vi "Close.vi"(11 "Custom Device Utility in":refnum<class "Custom Device Utility.lvclass">) -> (0 "error out":errorcluster, 3 "Custom Device Utility out":refnum<class "Custom Device Utility.lvclass">)   [LabVIEW 2027, in "Custom Device Interfaces.lvlib" / "Custom Device Utility.lvclass"]
uses:
  Custom Device Utility.lvclass
  Custom Device Utility.lvclass/Custom Device Utility.ctl
  CustomDevice/Custom Device.lvclass
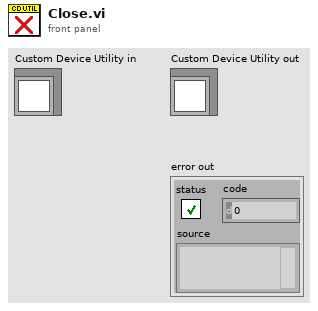
[diagram p1: front panel]
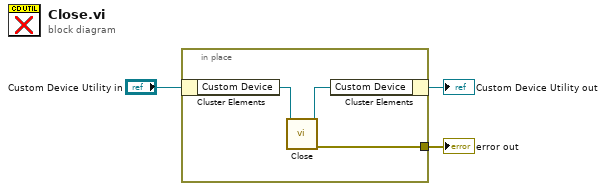
[diagram p0: block diagram]
diagram:
  n1 = in-place {
    in-place-border: [w6] -> w3
    n2 = in-place-cluster #1("Custom Device Utility in") -> ("Custom Device"=w5:refnum<class "Custom Device.lvclass">)
    n3 = call-dynamic "Close.vi"("Custom Device in"=w5) -> ("error out"=w6:errorcluster, "Custom Device out"=w4:refnum<class "Custom Device.lvclass">)  [unwired: 9 in]
    n4 = in-place-cluster #1("Custom Device"=w4) -> (→"Custom Device Utility out":refnum<class "Custom Device Utility.lvclass">)
  }
  "error out" <- w3
